vi "Current State.vi"() -> ()   [LabVIEW 2017]
uses:
  Type Definitions/Controller States.ctl
panel:
  in  "Controller States":T1
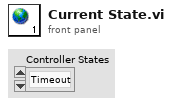
[diagram p1: front panel]
types:
  T1 = typedef "Controller States.ctl" = enum16{"Timeout", "Initial", "Login", "Idle", "Balance Inquiry", "Deposit", "Withdrawal", "Fast Cash", "Terminate", "Wait on Exit", "Shutdown", "Error Handler"}
diagram:
